vi "Boolean Crossing (DBL Array).vi"(2 "initialize":bool, 3 "direction":enum16{"either", "false-true", "true-false"}(ring), 5 "Input Booleans":bool[](array[boolean])) -> (1 "Crossings":bool[](array[boolean]))   [LabVIEW 2020, in "NI_AdvCtrl_nonlinear.lvlib"]
doc: "LabVIEW no longer supports this VI. You can obtain similar functionality by installing the LabVIEW Simulation Module.\n\nDetects boolean crossings of the input signal. The user can choose from three different detectors, either, minus-plus, and plus-minus."
uses:
  <vilib>/addons/control/advanced/NI_AdvCtrl_nonlinear.lvlib
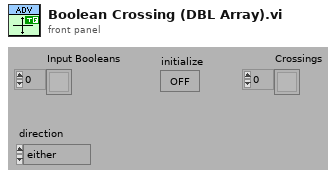
[diagram p1: front panel]
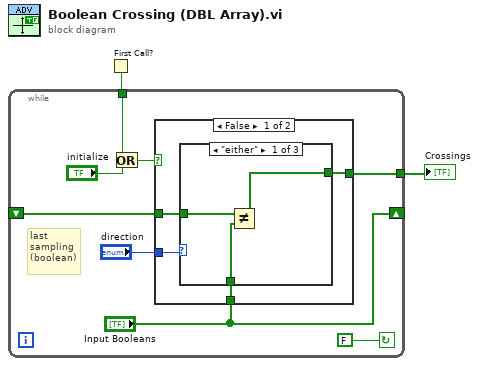
[diagram p0: block diagram]
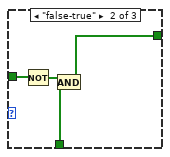
[diagram p2: hidden frame]
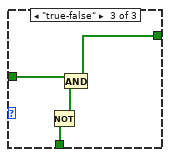
[diagram p3: hidden frame]
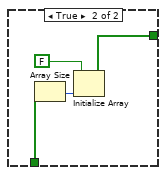
[diagram p4: hidden frame]
diagram:
  n1 = First Call?() -> (First Call?: T/F=w2:bool)
  n2 = while {
    tunnel: w2 -> [w5]
    tunnel: [w10] -> w1
    shift-left: _ -> [w8]
    shift-right: ["Input Booleans"] -> _
    stop <- FALSE continue-if-true
    # "last\nsampling\n(boolean)"
    n3 = Or(x=w5, y="initialize") -> (x .or. y?=w6:bool)
    n4 = case shown="False" w6 {
      tunnel: [w11 w26] -> w10
      tunnel: "direction" -> [w14 _]
      tunnel: w8 -> [w13 _]
      tunnel: "Input Booleans" -> [w12 w29]
      frame False {
        n5 = case shown="\"either\"" w14 {
          tunnel: w13 -> [w17 w20 w22]
          tunnel: w12 -> [w16 w18 w24]
          tunnel: [w15 w21 w25] -> w11
          frame "either" {
            n6 = Not Equal?(x=w17, y=w16) -> (x != y?=w15:bool[])
          }
          frame "false-true" {
            n7 = Not(x=w20) -> (.not. x?=w19:bool[])
            n8 = And(x=w19, y=w18) -> (x .and. y?=w21:bool[])
          }
          frame "true-false" {
            n9 = Not(x=w24) -> (.not. x?=w23:bool[])
            n10 = And(x=w22, y=w23) -> (x .and. y?=w25:bool[])
          }
        }
      }
      frame True {
        n11 = Array Size(array=w29) -> (size(s)=w28:i32)
        n12 = Initialize Array(FALSE, w28) -> (w26:bool[])
      }
    }
  }
  "Crossings" <- w1
